vi "myRIO__TCP_constants_port.vi"() -> (3 "output_TCP_port":u16=6340)   [LabVIEW 2014]
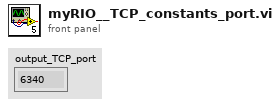
[diagram p1: front panel]
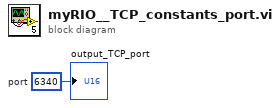
[diagram p0: block diagram]
diagram:
  w1 = u16 6340  # port
  "output_TCP_port" <- w1
